vi "DSF.Transceiver.GE Reflective Memory.Get GE 5565PIORC.vi"(11 "GE Reflective Memory in":refnum<class "DSF.Transceiver.GE Reflective Memory.lvclass">) -> (2 "GE 5565PIORC":refnum<class "GE 5565PIORC.lvclass">, 3 "GE Reflective Memory out":refnum<class "DSF.Transceiver.GE Reflective Memory.lvclass">)   [LabVIEW 2017, in "DSF.Transceiver.GE Reflective Memory.lvlib" / "DSF.Transceiver.GE Reflective Memory.lvclass"]
uses:
  DSF.Transceiver.GE Reflective Memory.lvclass
  C:/Git/DSF/DSF Core/Built/Engine/DSF.Engine.lvlibp/Engine/Classes/Transceiver/DSF.Engine.Transceiver.lvclass
  <vilib>/NI/GE Reflective Memory Driver/GE 5565PIORC.lvclass
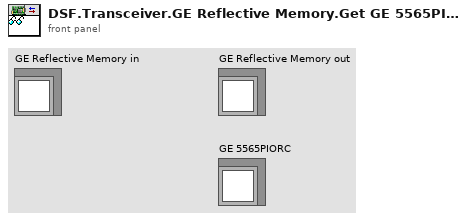
[diagram p1: front panel]
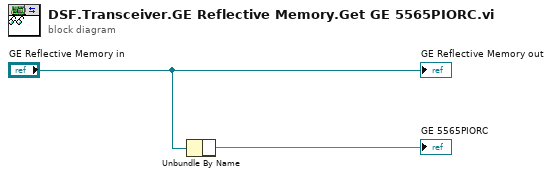
[diagram p0: block diagram]
diagram:
  n1 = Unbundle By Name("GE Reflective Memory in") -> (→"GE 5565PIORC")
  "GE Reflective Memory out" <- "GE Reflective Memory in"
